vi "HexCenterFinder4Points.vi"() -> ()   [LabVIEW 2019]
uses:
  <vilib>/userDefined/High Color/IMAQdx.ctl
panel:
  in  "YoffsetPCB":dbl format="%#_13g"
  in  "XoffsetPCB":dbl=166.649 format="%#_13g"
  in  "YoffsetSi":dbl format="%#_13g"
  in  "XoffsetSi":dbl format="%#_13g"
  in  "Position1?":bool=TRUE
  in  "Yoffset":dbl=0.05 format="%#_13g"
  out "yins":dbl[](array[numeric])
  out "Xins":dbl[](array[numeric])
  in  "Xoffset":dbl=165.962 format="%#_13g"
  in  "SiOnBP?":bool
  out "zAvg":dbl
  out "Output XYZU":string
  out "x":dbl
  out "y":dbl
  out "Orinetation":dbl
  in  "PCBEdges":path=path "C:/Users/TTUHEP/Documents/LabVIEW/Data/AssemblyIO_logs/PCB1_4Points.txt"
  in  "SiEdges":path=path "C:/Users/TTUHEP/Documents/LabVIEW/Data/AssemblyIO_logs/Si2Corners.txt"
  in  "Component":enum16{"Baseplate", "Si", "PCB"}(ring)
  in  "BasePlateEdges":path=path "C:/Users/TTUHEP/Documents/LabVIEW/Data/AssemblyIO_logs/Baseplate1CuPoints.txt"
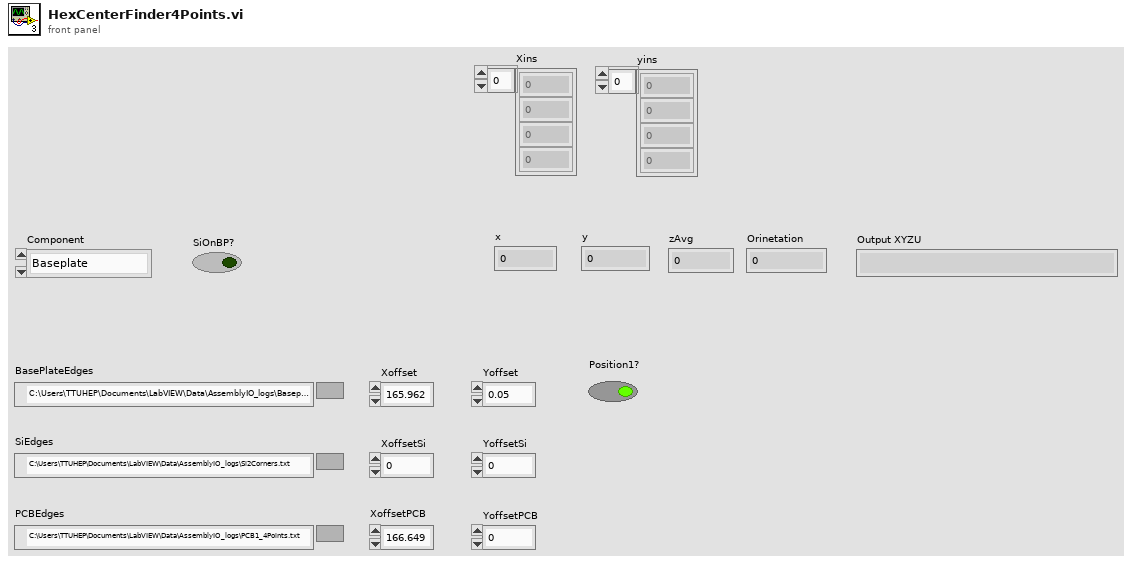
[diagram p1: front panel]
types:
  T1 = typedef "IMAQdx.ctl" = refnum<k21>
  T2 = typedef "IMAQ Image.ctl" = refnum<image>
  T3 = typedef "IMAQ Point" = cluster{"X":sgl, "Y":sgl}
  T4 = enum16{"Left Button", "Center Button", "Right Button", "Window Close"}
  T5 = enum16{"open", "replace", "create", "open or create", "replace or create", "replace or create with confirmation"}
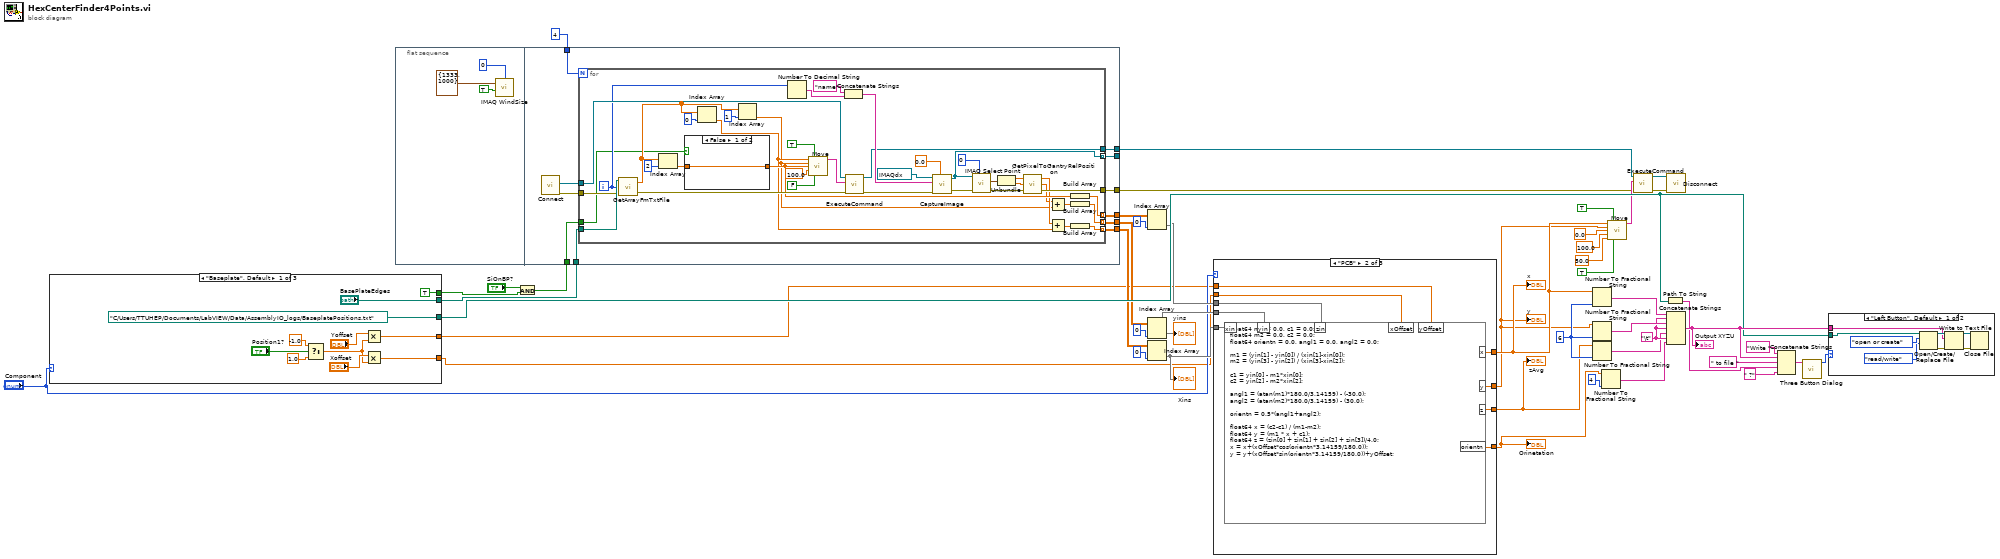
[diagram p0: block diagram]
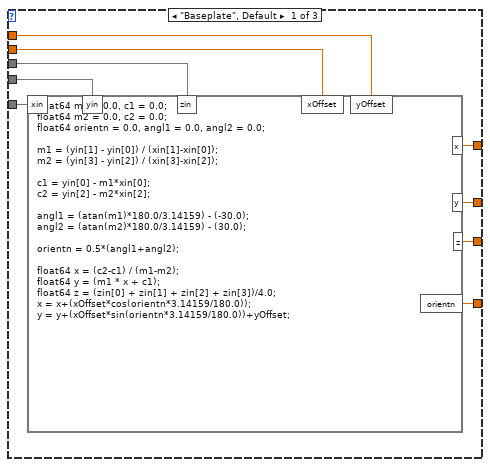
[diagram p2: hidden frame]
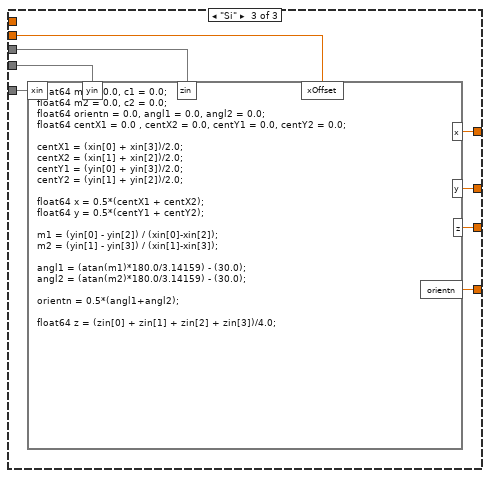
[diagram p3: hidden frame]
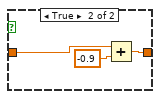
[diagram p5: hidden frame]
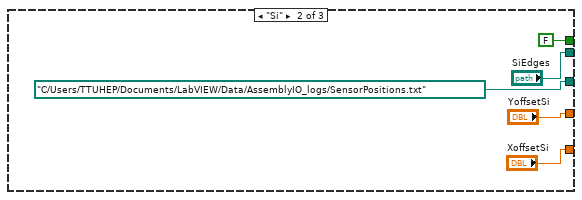
[diagram p6: hidden frame]
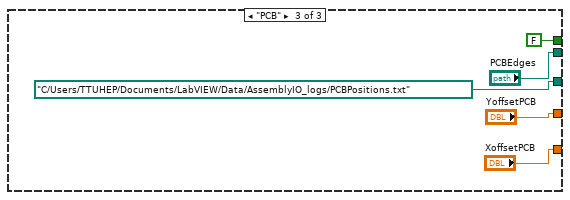
[diagram p7: hidden frame]
diagram:
  w42 = "\t"
  w39 = i16 6 ("width (-)")
  n1 = case shown="\"Baseplate\", Default" "Component" {
    tunnel: ["BasePlateEdges" "SiEdges" "PCBEdges"] -> w45
    tunnel: [path "C:/Users/TTUHEP/Documents/LabVIEW/Data/AssemblyIO_logs/BaseplatePositions.txt" ("OutFile") path "C:/Users/TTUHEP/Documents/LabVIEW/Data/AssemblyIO_logs/SensorPositions.txt" ("OutFile") path "C:/Users/TTUHEP/Documents/LabVIEW/Data/AssemblyIO_logs/PCBPositions.txt" ("OutFile")] -> w30
    tunnel: [TRUE ("y") FALSE ("y") FALSE ("y")] -> w29
    tunnel: [w48 "YoffsetSi" "YoffsetPCB"] -> w14
    tunnel: [w47 "XoffsetSi" "XoffsetPCB"] -> w13
    frame "Baseplate", Default {
      n2 = Select(t=-1.0, s="Position1?", f=1.0 ("t")) -> (s? t:f=w49:dbl)
      n3 = Multiply(x="Yoffset", y=w49) -> (x*y=w48:dbl)
      n4 = Multiply(x="Xoffset", y=w49) -> (x*y=w47:dbl)
    }
    frame "Si" {
    }
    frame "PCB" {
    }
  }
  n5 = flat-sequence {
    tunnel: 4 -> [w81]
    tunnel: w45 -> [w80]
    tunnel: [w79] -> w3
    tunnel: [w78] -> w5
    tunnel: [w75] -> _
    tunnel: [w74] -> w25
    tunnel: w27 -> [w73]
    tunnel: [w72] -> w21
    tunnel: [w71] -> w23
    frame #0 {
      n6 = call "IMAQ WindSize"("Scrollbars? (N)"=TRUE, "Width & Height"=cluster{"Width":i32, "Height":i32} {"Width"=1333, "Height"=1000}, "Window Number"=0) -> ()  [unwired: 3 in, 3 out]
    }
    frame #1 {
      n7 = call "Connect.vi"() -> ("error out"=w77:errorcluster, "controller"=w76:refnum<k24>)  [unwired: 10 in]
      n8 = for {
        N: w81 -> [_]
        tunnel: w80 -> [w117]
        tunnel: w76 -> [w109]
        tunnel: w77 -> [w108]
        tunnel: [w92] -> w79
        tunnel: [w93] -> w78
        tunnel: [w102] -> w75 mode=indexing
        tunnel: [w101] -> w74 mode=indexing
        tunnel: w73 -> [w100]
        tunnel: [w91] -> w72 mode=indexing
        tunnel: [w90] -> w71 mode=indexing
        i -> [w106]
        n9 = call "GetArrayFmTxtFile.vi"("error in"=w108, "LineNo."=w106, "TextFile"=w117) -> ("error out"=w107:errorcluster, "Array"=w118:dbl[])
        n10 = Index Array(array=w118, index=2) -> (element=w99:dbl)
        n11 = case shown="False" w100 {
          tunnel: w99 -> [w122 w125]
          tunnel: [w122 w123] -> w98
          frame False {
          }
          frame True {
            n12 = Add(x=w125, y=-0.9) -> (x+y=w123:dbl)
          }
        }
        n13 = Index Array(array=w118, index=0) -> (element=w88:dbl)
        n14 = Index Array(array=w118, index=1) -> (element=w86:dbl)
        n15 = Number To Decimal String(number=w106) -> (decimal integer string=w105:string)  [unwired: 1 in]
        n16 = call "Move.vi"("X"=w88, "Absolute"=TRUE, "Y"=w86, "Z"=w98, "SpeedXY (mm/s)"=100.0, "Move Z first"=FALSE) -> ("Position Gcode"=w110:string)  [unwired: 9 in]
        n17 = Concatenate Strings("name" ("string"), w105) -> (w103:string)
        n18 = call "ExecuteCommand.vi"("error in (no error)"=w107, "Command Code"=w110, "controller in"=w109) -> ("error out"=w113:errorcluster, "controller out"=w93:refnum<k24>)  [unwired: 6 in, 1 out]
        n19 = call "CaptureImage.vi"("Camera"=T1 "cam0", "Rotate (degrees)"=sgl 0.0, "ImageName"=w103, "error in (no error)"=w113) -> ("Image"=w102:T2, "error out"=w111:errorcluster)  [unwired: 3 in]
        n20 = call "IMAQ Select Point"("Window Number (0...15)"=0, "error in (no error)"=w111, "Image In"=w102) -> ("error out"=w94:errorcluster, "Point"=w97:T3)  [unwired: 5 in, 2 out]
        n21 = Unbundle(w97) -> ("X"=w96:sgl, "Y"=w95:sgl)
        n22 = call "GetPixelToGantryRelPosition.vi"("error in (no error)"=w94, "PixelY"=w95, "PixelX"=w96) -> ("error out"=w92:errorcluster, "YmmRelGH"=w85:dbl, "XmmRelGH"=w89:dbl)
        n23 = Add(x=w85, y=w86) -> (x+y=w84:dbl)
        n24 = Add(x=w89, y=w88) -> (x+y=w87:dbl)
        n25 = Build Array(w98) -> (w101:dbl[])
        n26 = Build Array(w84) -> (w91:dbl[])
        n27 = Build Array(w87) -> (w90:dbl[])
      }
    }
  }
  n28 = And(x="SiOnBP?", y=w29) -> (x .and. y?=w27:bool)
  n29 = Index Array(array=w25, index (col)=0 ("disabled index (col)")) -> (element=w18:dbl[])  [unwired: 1 in]
  n30 = Index Array(array=w21, index (col)=0 ("disabled index (col)")) -> (element=w19:dbl[])  [unwired: 1 in]
  "yins" <- w19
  n31 = Index Array(array=w23, index (col)=0 ("disabled index (col)")) -> (element=w20:dbl[])  [unwired: 1 in]
  "Xins" <- w20
  n32 = case shown="\"PCB\"" "Component" {
    tunnel: w20 -> [w134 w143 w151]
    tunnel: w19 -> [w133 w142 w150]
    tunnel: w18 -> [w132 w141 w149]
    tunnel: w13 -> [w131 w140 w148]
    tunnel: [w130 w139 w147] -> w17
    tunnel: [w129 w138 w146] -> w12
    tunnel: [w128 w137 w145] -> w11
    tunnel: [w127 w136 w144] -> w16
    tunnel: w14 -> [w126 w135 _]
    frame "Baseplate", Default {
      n33 = formula code="float64 m1 = 0.0, c1 = 0.0;\nfloat64 m2 = 0.0, c2 = 0.0;\nfloat64 orientn = 0.0, angl1 = 0.0, angl2 = 0.0;\n\nm1 = (yin[1] - yin[0]) / (xin[1]-xin[0]);\nm2 = (yin[3] - yin[2]) / (xin[3]-xin[2]);\n\nc1 = yin[0] - m1*xin[0];\nc2 = yin[2] - m2*xin[2];\n\nangl1 = (atan(m1)*180.0/3.14159) - (-30.0);\nangl2 = (atan(m2)*180.0/3.14159) - (30.0);\n\norientn = 0.5*(angl1+angl2);\n\nfloat64 x = (c2-c1) / (m1-m2);\nfloat64 y = (m1 * x + c1);\nfloat64 z = (zin[0] + zin[1] + zin[2] + zin[3])/4.0;\nx = x+(xOffset*cos(orientn*3.14159/180.0));\ny = y+(xOffset*sin(orientn*3.14159/180.0))+yOffset;"("xin"=w134, "yin"=w133, "zin"=w132, "xOffset"=w131, "yOffset"=w126) -> ("orientn"=w130:dbl, "x"=w129:dbl, "y"=w128:dbl, "z"=w127:dbl)
    }
    frame "PCB" {
      n34 = formula code="float64 m1 = 0.0, c1 = 0.0;\nfloat64 m2 = 0.0, c2 = 0.0;\nfloat64 orientn = 0.0, angl1 = 0.0, angl2 = 0.0;\n\nm1 = (yin[1] - yin[0]) / (xin[1]-xin[0]);\nm2 = (yin[3] - yin[2]) / (xin[3]-xin[2]);\n\nc1 = yin[0] - m1*xin[0];\nc2 = yin[2] - m2*xin[2];\n\nangl1 = (atan(m1)*180.0/3.14159) - (-30.0);\nangl2 = (atan(m2)*180.0/3.14159) - (30.0);\n\norientn = 0.5*(angl1+angl2);\n\nfloat64 x = (c2-c1) / (m1-m2);\nfloat64 y = (m1 * x + c1);\nfloat64 z = (zin[0] + zin[1] + zin[2] + zin[3])/4.0;\nx = x+(xOffset*cos(orientn*3.14159/180.0));\ny = y+(xOffset*sin(orientn*3.14159/180.0))+yOffset;"("xin"=w143, "yin"=w142, "zin"=w141, "xOffset"=w140, "yOffset"=w135) -> ("orientn"=w139:dbl, "x"=w138:dbl, "y"=w137:dbl, "z"=w136:dbl)
    }
    frame "Si" {
      n35 = formula code="float64 m1 = 0.0, c1 = 0.0;\nfloat64 m2 = 0.0, c2 = 0.0;\nfloat64 orientn = 0.0, angl1 = 0.0, angl2 = 0.0;\nfloat64 centX1 = 0.0 , centX2 = 0.0, centY1 = 0.0, centY2 = 0.0;\n\ncentX1 = (xin[0] + xin[3])/2.0;\ncentX2 = (xin[1] + xin[2])/2.0;\ncentY1 = (yin[0] + yin[3])/2.0;\ncentY2 = (yin[1] + yin[2])/2.0;\n\nfloat64 x = 0.5*(centX1 + centX2); \nfloat64 y = 0.5*(centY1 + centY2);\n\nm1 = (yin[0] - yin[2]) / (xin[0]-xin[2]);\nm2 = (yin[1] - yin[3]) / (xin[1]-xin[3]);\n\nangl1 = (atan(m1)*180.0/3.14159) - (30.0);\nangl2 = (atan(m2)*180.0/3.14159) - (30.0);\n\norientn = 0.5*(angl1+angl2);\n\nfloat64 z = (zin[0] + zin[1] + zin[2] + zin[3])/4.0;"("xin"=w151, "yin"=w150, "zin"=w149, "xOffset"=w148) -> ("orientn"=w147:dbl, "x"=w146:dbl, "y"=w145:dbl, "z"=w144:dbl)
    }
  }
  "Orinetation" <- w17
  "y" <- w11
  "x" <- w12
  "zAvg" <- w16
  n36 = Number To Fractional String(number=w12, precision (6)=w39) -> (F-format string=w44:string)  [unwired: 2 in]
  n37 = Number To Fractional String(number=w11, precision (6)=w39) -> (F-format string=w43:string)  [unwired: 2 in]
  n38 = Number To Fractional String(number=w16, precision (6)=w39) -> (F-format string=w38:string)  [unwired: 2 in]
  n39 = Number To Fractional String(number=w17, precision (6)=i16 4 ("width (-)")) -> (F-format string=w40:string)  [unwired: 2 in]
  n40 = call "Move.vi"("X"=w12, "Absolute"=TRUE, "Y"=w11, "Z"=0.0, "SpeedXY (mm/s)"=100.0, "SpeedZ (mm/s)"=50.0, "Move Z first"=TRUE) -> ("Position Gcode"=w4:string)  [unwired: 8 in]
  n41 = call "ExecuteCommand.vi"("error in (no error)"=w3, "Command Code"=w4, "controller in"=w5) -> ("error out"=w2:errorcluster, "controller out"=w1:refnum<k24>)  [unwired: 6 in, 1 out]
  n42 = Path To String(path=w30) -> (string=w34:string)
  n43 = call "Disconnect.vi"("error in (no error)"=w2, "controller"=w1) -> ()  [unwired: 9 in, 1 out]
  n44 = Concatenate Strings(w44, w42, w43, w42, w38, w42, w40) -> (w36:string)
  "Output XYZU" <- w36
  n45 = Concatenate Strings("Write ", w36, " to file ", w34, " ?" ("string")) -> (w32:string)
  n46 = call <vilib>:"Three Button Dialog.vi"("message"=w32) -> ("Which Button?"=w31:T4)  [unwired: 10 in]
  n47 = case shown="\"Left Button\", Default" w31 {
    tunnel: w36 -> [w153 _]
    tunnel: w30 -> [w152 _]
    frame "Left Button", Default {
      n48 = Open/Create/Replace File(file path (use dialog)=w152, operation (0:open)=T5."open or create", access (0:read/write)=enum16{"read/write", "read-only", "write-only"}."read/write") -> (refnum out=w159:refnum<file>, error out=w156:errorcluster)  [unwired: 3 in, 1 out]
      n49 = Write to Text File(file (use dialog)=w159, text=w153, error in=w156) -> (refnum out=w154:refnum<file>, error out=w155:errorcluster)  [unwired: 1 in, 1 out]
      n50 = Close File(refnum=w154, error in=w155) -> ()  [unwired: 2 out]
    }
    frame "Center Button" {
    }
  }
